vi "Turn on an ARC.vi"(0 "Change in Gyro (deg)":dbl, 1 "Radius(t) or arc length(f)":dbl, 2 "Measurement Mode":bool, 3 "error in (no error)":errorcluster) -> (10 "error out":errorcluster)   [LabVIEW 2017]
uses:
  <vilib>/Rock Robotics/WPI/ThirdParty/Sensors/navX/_TypeDefs/FRIC_navX_DeviceNumbersTypeDef.ctl
  <vilib>/Rock Robotics/WPI/ThirdParty/Phoenix-LabVIEW/Motor Controller/Get/CTRE_Phoenix_MotorController_GetSelectedSensorData.vi
  <vilib>/Rock Robotics/WPI/ThirdParty/Phoenix-LabVIEW/Motor Controller/Controls/CTRE_Phoenix_MotorControl_FeedbackDevice.ctl
panel:
  # "no idea if this will work\nmight make a radius twice as big as inputed"
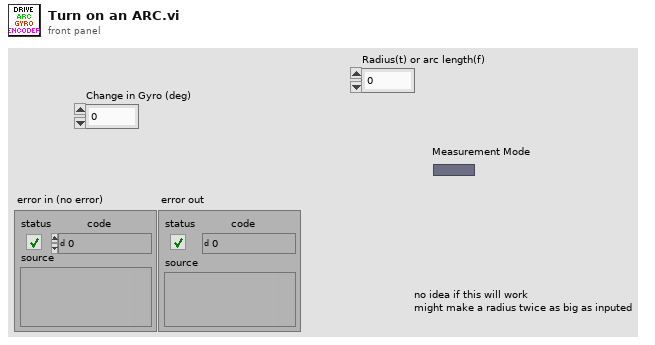
[diagram p1: front panel]
types:
  T1 = typedef "CTRE_Phoenix_MotorControl_FeedbackDevice.ctl" = i8
  T2 = typedef "FRIC_navX_DeviceNumbersTypeDef.ctl" = enum16{"Dev0", "Dev1", "Dev2", "Dev3"}
  T3 = typedef "WPI_MotorControlDeviceRef.ctl" = cluster{"DeviceStatus":errorcluster, "Type":T4, "PWM":cluster{"PWM Channel":T5, "DeadBand":T6}, "CAN":cluster{"Device Number":u8, "SetOutput VI Ref":variant, "GetOutput VI Ref":variant, "Enable VI Ref":variant, "Disable VI Ref":variant, "Data":variant}, "Invert":bool, "DIO PWM":cluster{"PWM \"Enable\" Channel":T5, "DIOChannel":T7, "PWM Rate":dbl}}
  T4 = typedef "WPI_MotorControlType.ctl" = enum16{"PWM", "CAN", "DIO PWM"}
  T5 = typedef "FPGA_DIOPWMChannel.ctl" = enum8{"PWM 0", "PWM 1", "PWM 2", "PWM 3", "PWM 4", "PWM 5", "PWM 6", "PWM 7", "PWM 8", "PWM 9", "PWM MXP 0", "PWM MXP 1", "PWM MXP 2", "PWM MXP 3", "PWM MXP 4", "PWM MXP 5", "PWM MXP 6", "PWM MXP 7", "PWM MXP 8", "PWM MXP 9", "Invalid"}
  T6 = typedef "WPI_PWMDeadband.ctl" = cluster{"Name":string, "maxPositivePwm":i32, "minPositivePwm":i32, "centerPwm":i32, "maxNegativePwm":i32, "minNegativePwm":i32, "angularRange":u16}
  T7 = typedef "FPGA_DIOChannel.ctl" = enum8{"DIO 0", "DIO 1", "DIO 2", "DIO 3", "DIO 4", "DIO 5", "DIO 6", "DIO 7", "DIO 8", "DIO 9", "DIO MXP 0", "DIO MXP 1", "DIO MXP 2", "DIO MXP 3", "DIO MXP 4", "DIO MXP 5", "DIO MXP 6", "DIO MXP 7", "DIO MXP 8", "DIO MXP 9", "DIO MXP 10", "DIO MXP 11", "DIO MXP 12", "DIO MXP 13", "DIO MXP 14", "DIO MXP 15", "SPI Port CS1", "SPI Port CS2", "SPI Port CS3", "SPI Port MISO", "SPI Port MOSI", "Invalid"}
  T8 = cluster{"Yaw":dbl, "Roll":dbl, "Pitch":dbl, "Heading":dbl, "Fused Heading":dbl}
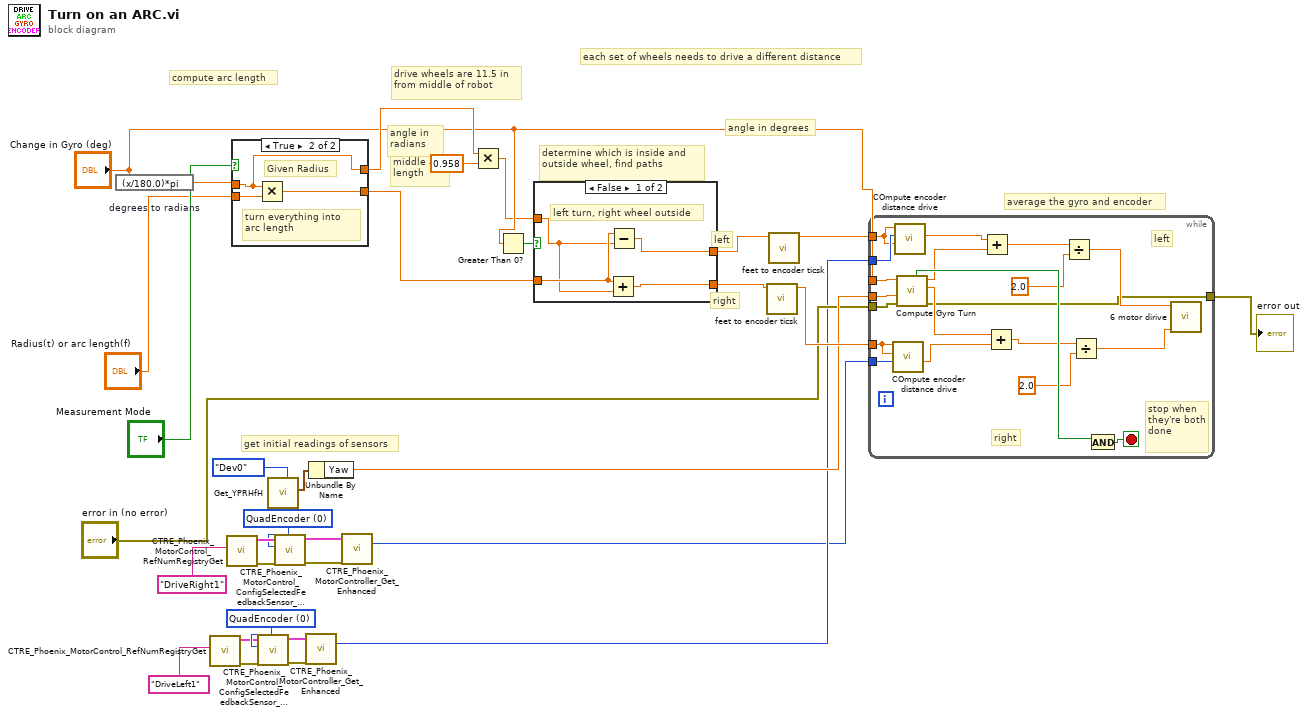
[diagram p0: block diagram]
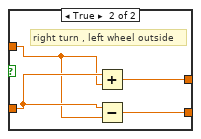
[diagram p2: hidden frame]
diagram:
  w17 = T1 0 items=["None"=-1, "QuadEncoder"=0, "Analog"=2, "Tachometer"=4, "Pulse Width Encoded Position"=8, "Sensor Sum (S0 + S1)"=9, "Sensor Difference (D0 - D1)"=10, "Remote Source 0"=11, "Remote Source 1"=12, "Software Emulated"=15] ("Feedback Device")
  w24 = T1 0 items=["None"=-1, "QuadEncoder"=0, "Analog"=2, "Tachometer"=4, "Pulse Width Encoded Position"=8, "Sensor Sum (S0 + S1)"=9, "Sensor Difference (D0 - D1)"=10, "Remote Source 0"=11, "Remote Source 1"=12, "Software Emulated"=15] ("Feedback Device")
  # "average the gyro and encoder"
  # "left"
  # "right"
  # "determine which is inside and outside wheel, find paths"
  # "each set of wheels needs to drive a different distance"
  # "drive wheels are 11.5 in from middle of robot"
  # "angle in degrees"
  # "angle in radians"
  # "get initial readings of sensors"
  # "compute arc length"
  # "middle arc length"
  n1 = expression code="(x/180.0)*pi" "degrees to radians"("Change in Gyro (deg)") -> (w13:dbl)
  n2 = call <vilib>:"CTRE_Phoenix_MotorControl_RefNumRegistryGet.vi"("refnum name"="DriveLeft1") -> ("error out"=w19:errorcluster, "PhoenixMotorControlDevRef"=w16:T3)  [unwired: 9 in]
  n3 = call <vilib>:"CTRE_Phoenix_MotorControl_RefNumRegistryGet.vi"("refnum name"="DriveRight1") -> ("error out"=w22:errorcluster, "PhoenixMotorControlDevRef"=w25:T3)  [unwired: 9 in]
  n4 = case shown="True" "Measurement Mode" {
    tunnel: "Radius(t) or arc length(f)" -> [w34 w35]
    tunnel: [w34 w37] -> w7
    tunnel: w13 -> [w33 w36]
    tunnel: [w33 w36] -> w12
    frame False {
      # "Given Arc Length"
    }
    frame True {
      # "turn everything into arc length"
      # "Given Radius"
      n5 = Multiply(x=w36, y=w35) -> (x*y=w37:dbl)
    }
  }
  n6 = call <vilib>:"CTRE_Phoenix_MotorControl_ConfigSelectedFeedbackSensor_Enhanced.vi"("error in (no error)"=w19, "Feedback Device"=w17, "PhoenixMotorControlDevRef"=w16) -> ("error out"=w20:errorcluster, "PhoenixMotorControlDevRef"=w15:T3)  [unwired: 7 in]
  n7 = call <vilib>:"Get_YPRHfH.vi"("Device Number"=FRIC_navX_DeviceNumbersTypeDef."Dev0") -> ("YRPHfH"=w29:T8)  [unwired: 10 in]
  n8 = call <vilib>:"CTRE_Phoenix_MotorControl_ConfigSelectedFeedbackSensor_Enhanced.vi"("error in (no error)"=w22, "Feedback Device"=w24, "PhoenixMotorControlDevRef"=w25) -> ("error out"=w21:errorcluster, "PhoenixMotorControlDevRef"=w26:T3)  [unwired: 7 in]
  n9 = call-poly <vilib>:"CTRE_Phoenix_MotorController_Get_Enhanced.vi"("PhoenixMotorControlDevRef"=w15, "error in"=w20) -> ("Position (Raw Sensor Units)"=w3:i32)  [unwired: 10 in, 3 out]
  n10 = Unbundle By Name(w29) -> ("Yaw"=w27:dbl)
  n11 = call-poly <vilib>:"CTRE_Phoenix_MotorController_Get_Enhanced.vi"("PhoenixMotorControlDevRef"=w26, "error in"=w21) -> ("Position (Raw Sensor Units)"=w2:i32)  [unwired: 10 in, 3 out]
  n12 = Multiply(x=w12, y=0.958) -> (x*y=w8:dbl)
  n13 = Greater Than 0?(x="Change in Gyro (deg)") -> (x > 0?=w10:bool)
  n14 = case shown="False" w10 {
    tunnel: w8 -> [w40 w44]
    tunnel: w7 -> [w41 w45]
    tunnel: [w39 w43] -> w6
    tunnel: [w38 w42] -> w5
    frame False {
      # "left turn, right wheel outside"
      n15 = Add(x=w41, y=w40) -> (x+y=w38:dbl)
      n16 = Subtract(x=w41, y=w40) -> (x-y=w39:dbl)
    }
    frame True {
      # "right turn , left wheel outside"
      n17 = Add(x=w45, y=w44) -> (x+y=w43:dbl)
      n18 = Subtract(x=w45, y=w44) -> (x-y=w42:dbl)
    }
  }
  n19 = call "feet to encoder ticsk.vi"("Distance in feet wanted"=w5) -> ("Encoder Ticks"=w30:dbl)  [unwired: 10 in]
  n20 = call "feet to encoder ticsk.vi"("Distance in feet wanted"=w6) -> ("Encoder Ticks"=w4:dbl)  [unwired: 10 in]
  n21 = while {
    tunnel: w30 -> [w58]
    tunnel: "Change in Gyro (deg)" -> [w65]
    tunnel: w27 -> [w64]
    tunnel: "error in (no error)" -> [w61]
    tunnel: w4 -> [w59]
    tunnel: w3 -> [w60]
    tunnel: w2 -> [w57]
    tunnel: [w46] -> w1
    stop <- w63 stop-if-true
    # "right"
    # "left"
    # "stop when they're both done"
    n22 = call "COmpute encoder distance drive.vi"("Right Starting"=w57, "Left Starting"=w58, "Wanted Distance"=w58) -> ("Right Drive"=w53:dbl)  [unwired: 5 in, 3 out]
    n23 = call "COmpute encoder distance drive.vi"("Right Starting"=w59, "Left Starting"=w60, "Wanted Distance"=w59) -> ("Left Drive"=w56:dbl)  [unwired: 5 in, 3 out]
    n24 = call "Compute Gyro Turn.vi"("error in (no error)"=w61, "Starting Degree"=w64, "Turn? Right Positive."=w65) -> ("error out"=w46:errorcluster, "Right Drive"=w54:dbl, "Left drive"=w55:dbl, "done"=w62:bool)  [unwired: 5 in]
    n25 = Add(x=w56, y=w55) -> (x+y=w51:dbl)
    n26 = Add(x=w54, y=w53) -> (x+y=w49:dbl)
    n27 = Divide(x=w51, y=2.0) -> (x/y=w47:dbl)
    n28 = Divide(x=w49, y=2.0) -> (x/y=w48:dbl)
    n29 = And(x=w62) -> (x .and. y?=w63:bool)  [unwired: 1 in]
    n30 = call "6 motor dirive.vi"("Right Joystick"=w48, "Left Joystick"=w47) -> ()  [unwired: 10 in]
  }
  "error out" <- w1
